vi "RGBimg2bin2RGBimg.vi"() -> ()   [LabVIEW 2018, in "LabView-0mq-Jl_Roundtrip_lib.lvlib"]
uses:
  LabView-0mq-Jl_Roundtrip_lib.lvlib
panel:
  out "error out":errorcluster
  in  "peppers":bool
  in  "Path":path=path "C:/_MyOwnDocs/MyTmp/ScreenShots/2019-07-30 14_38_29-Desktop Execution Trace Toolkit.png"
  out "picture dup":picture
  out "picture":picture
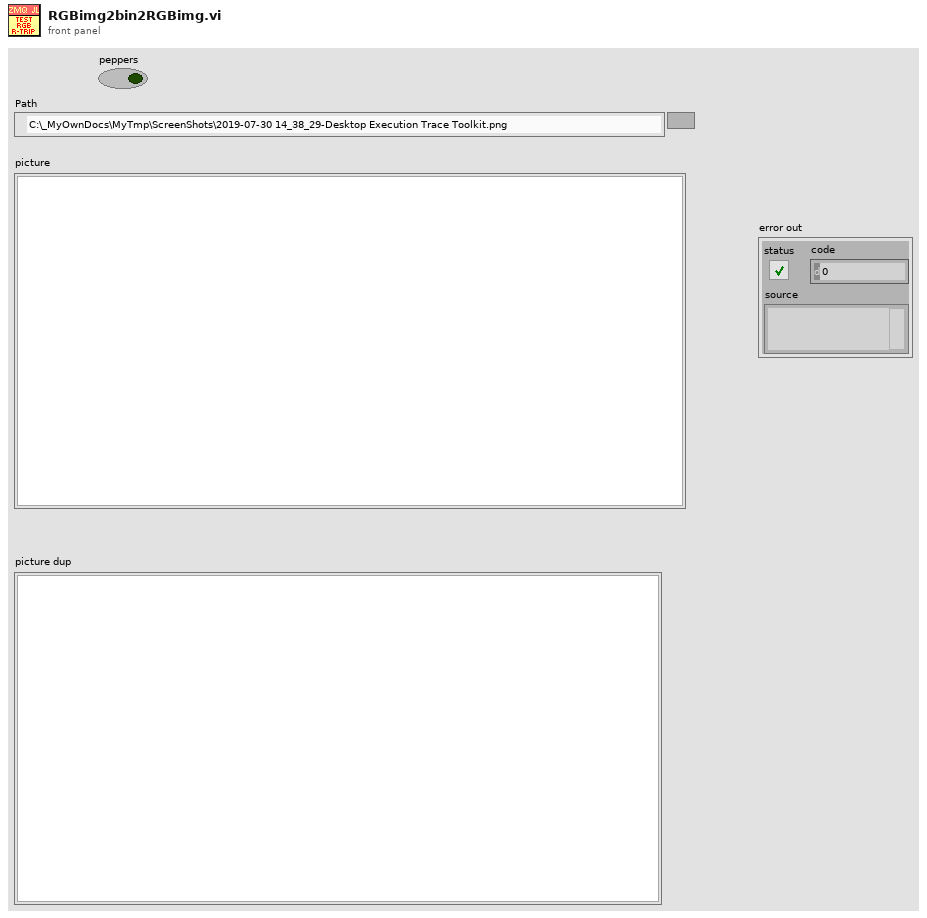
[diagram p1: front panel]
types:
  T1 = typedef "imagedata.ctl" = cluster{"image type":i32, "image depth":i32, "image":u8[], "mask":u8[], "colors":u32[], "Rectangle":cluster{"left":i16, "top":i16, "right":i16, "bottom":i16}}
  T2 = typedef "Bindata&description.ctl" = cluster{"bindata_descr":T3[], "bindata":u8[]}
  T3 = typedef "LabView-0mq-Jl_Roundtrip_lib.lvlib/Bindata description.ctl" = cluster{"nofbytes":i32, "numtype":string, "start":i32, "arrdims":i32[], "kwarg_name":string, "category":string}
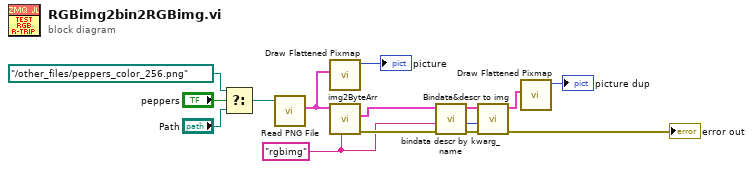
[diagram p0: block diagram]
diagram:
  w1 = "rgbimg" ("Tag")
  n1 = Select(t=path "../other_files/peppers_color_256.png" ("Path"), s="peppers", f="Path") -> (s? t:f=w8:path)
  n2 = call <vilib>:"Read PNG File.vi"("path to PNG file"=w8) -> ("image data"=w14:T1)  [unwired: 8 in, 2 out]
  n3 = call <vilib>:"Draw Flattened Pixmap.vi"("image data"=w14) -> ("new picture"=→"picture":picture)  [unwired: 8 in]
  n4 = call "img2ByteArr.vi"("kwarg_name"=w1, "img in"=w14) -> ("error out"=w6:errorcluster, "Bindata & descr out"=w4:T2)  [unwired: 7 in, 1 out]
  n5 = call "bindata descr by kwarg_name.vi"("Error in"=w6, "kwarg_name"=w1, "Bindata & descr"=w4) -> ("Error out"=w5:errorcluster, "index"=w2:i32, "Bindata & descr out"=w3:cluster{"bindata_descr":T3[], "bindata":u8[]})  [unwired: 5 in, 1 out]
  n6 = call "Bindata&descr to img.vi"("error in (no error)"=w5, "bindata_descr index"=w2, "Bindata & descr in"=w3) -> ("error out"=→"error out":errorcluster, "img out"=w13:T1)  [unwired: 7 in]
  n7 = call <vilib>:"Draw Flattened Pixmap.vi"("image data"=w13) -> ("new picture"=→"picture dup":picture)  [unwired: 8 in]
